vi "ImagerForFlowbit3.vi"() -> ()   [LabVIEW 2011]
uses:
  <vilib>/vision/Image Controls.llb/IMAQ Image.ctl
  <vilib>/Platform/TimedLoop/XDataNode/timing_clust.ctl
  <vilib>/Platform/TimedLoop/XDataNode/nitl_modes.ctl
  <vilib>/Platform/TimedLoop/XDataNode/wakeup.ctl
  <vilib>/Analysis/1siggen.llb/Riffle Array (I32).vi
  <vilib>/Platform/TimedLoop/XDataNode/XDataNode.xnode
  <vilib>/Analysis/NI_AALBase.lvlib
  <vilib>/vision/NI_Vision_Development_Module.lvlib
  <vilib>/Platform/TimedLoop/XDataNode/XDNodeRunTimeDep.lvlib
panel:
  out "数组 2":bool[](array[boolean])
  out "OnlineMap Array":T1[](array[typedef])
  out "DR/R array":T1[](array[typedef])
  out "停止循环":bool
  in  "Stimuli":i64=5
  in  "FrameHeight":i64=576
  in  "FrameWidth":i64=704
  in  "选项卡控件":enum32{"前面板", "参数设置", "OnLineMap"}(tab)
  out "log":string
  out "Stim_ID":i32(listbox)=1
  in  "开始/暂停":bool=TRUE
  in  "停止":bool
  out "重排的 Stim ID":i32[](array[numeric]) caption="重排的{X}"
  out "block":i32
  out "队列中元素数量":i32
  out "Image 2":T1(plugin-control)
  in  "热图":bool
  out "循环持续时间":i64
  out "Recording":bool
  in  "FramesPerStim(100Hz)":i64=16
  in  "Blk目录":path=path "D:/Expt/test"
  in  "文件名":string="G4_E01"
  in  "TimeForPrepare(ms)":u32=1000
  in  "stim ID":u8[](array[numeric])=[0, 2, 4, 6, 8]
  in  "blk总数":i32=500
  in  "stim protocol":T2(array[ring])=[enum."prep stim", enum."wait respirator", enum."show stim", enum."recording data", enum."Blank stim", enum."ISI"]
  in  "blank stim":u8
  in  "wait（ms）":u32=10
  in  "ISI（ms）":u32=8000
  in  "FrameBin":i32=25
  in  "datatype":u16(ring)=13 items=["U8"=11, "I16"=12, "U32"=13, "SGL"=14]
  in  "OnlineMap":cluster{"数组 1":i32[], "数组 2":i32[]}[](array[cluster])=[{"数组 1"=[2], "数组 2"=[6]}, {"数组 1"=[4], "数组 2"=[8]}, {"数组 1"=[2, 6], "数组 2"=[4, 8]}, {"数组 1"=[2, 4, 6, 8], "数组 2"=[0]}, {"数组 1"=[2, 4], "数组 2"=[6, 8]}]
  in  "DR/R parameter":T3={"frame_zero_0"=0, "frame_zero_1"=1, "frame_0"=3, "frame_1"=15}
  # "÷"
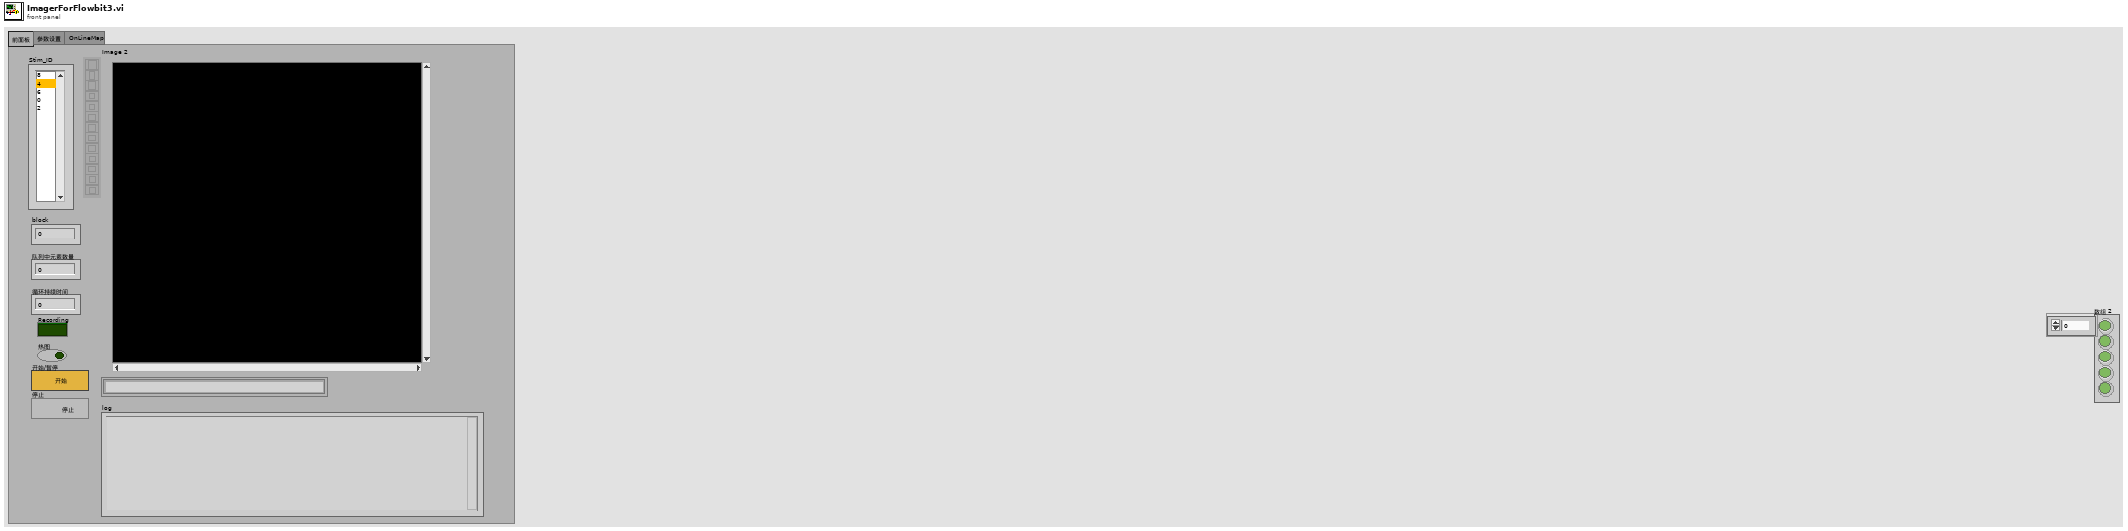
[diagram p1: front panel]
types:
  T1 = typedef "IMAQ Image.ctl" = refnum<image>
  T2 = enum16{"wait", "prep stim", "show stim", "wait respirator", "recording data", "Blank stim", "wait heart", "ISI", "DR/R", "wait calibrate"}[]
  T3 = cluster{"frame_zero_0":i32, "frame_zero_1":i32, "frame_0":i32, "frame_1":i32}
  T4 = typedef "Image Type" = u32
  T5 = enum16{"Disable External Trigger", "Enable External Trigger"}
  T6 = enum32{"Auto Detect", "RoadRunner", "Raven", "R64"}
  T7 = typedef "XDNodeRunTimeDep.lvlib/timing_clust.ctl" = cluster{"Expected End [f-1]":u64, "Actual End [f-1]":u64, "Finished Late? [f-1]":bool, "Expected End [i-1]":u64, "Actual End [i-1]":u64, "Finished Late? [i-1]":bool, "Expected Start [i]":u64, "Actual Start [i]":u64, "Expected Start [f]":u64, "Actual Start [f]":u64, "Source Name":string, "Structure Name":string, "Period":i64, "Deadline":i64, "Offset":i64, "Start":i64, "Priority":i32, "Timeout":i32, "Mode":T8, "Wakeup Reason":T9, "Error":errorcluster, "Source Type":string, "Secondary Source Type":string, "Global End Time":u64, "Global Start Time":u64, "Frame Duration":u64, "Iteration Duration":u64, "Assigned CPU":i32, "I/O Scan Engine Mode":u32}
  T8 = typedef "XDNodeRunTimeDep.lvlib/nitl_modes.ctl" = enum32{"No Change", "Process missed periods, maintain original phase", "Discard missed periods, maintain original phase", "Process missed periods, ignore original phase", "Discard missed periods, ignore original phase"}
  T9 = typedef "XDNodeRunTimeDep.lvlib/wakeup.ctl" = enum32{"Normal", "Aborted", "Asynchronous wakeup", "Timing source error", "Timed loop error", "Timeout"}
  T10 = enum16{"big-endian, network order", "native, host order", "little-endian"}
  T11 = enum16{"open", "replace", "create", "open or create", "replace or create", "replace or create with confirmation"}
  T12 = cluster{"Mean Value":sgl, "Standard Variation":sgl, "Minimal Value":sgl, "Maximal Value":sgl, "Area (calibrated)":sgl, "Area (pixels)":u32, "%":sgl, "Calibration Valid":bool}
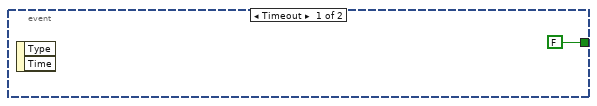
[diagram p2: hidden frame]
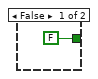
[diagram p3: hidden frame]
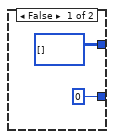
[diagram p5: hidden frame]
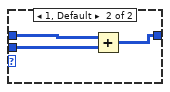
[diagram p7: hidden frame]
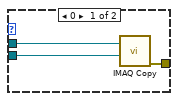
[diagram p8: hidden frame]
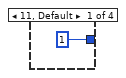
[diagram p9: hidden frame]
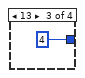
[diagram p10: hidden frame]
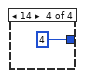
[diagram p11: hidden frame]
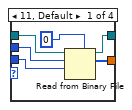
[diagram p12: hidden frame]
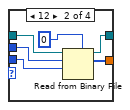
[diagram p13: hidden frame]
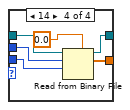
[diagram p14: hidden frame]
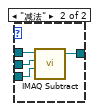
[diagram p18: hidden frame]
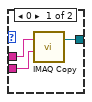
[diagram p19: hidden frame]
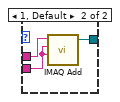
[diagram p20: hidden frame]
diagram:
  w1 = u32[][] []
  w14 = T4 4 items=["Grayscale (U8)", "Grayscale (I16)", "Grayscale (SGL)", "Complex (CSG)", "RGB (U32)", "HSL (U32)", "RGB (U64)", "Grayscale (U16)"] ("Image Type")
  w12 = u32[] [160, 240, 2105599, 873983, 50382, 65535, 65344, 8454016, 16776960, 16777088, 16744512, 16711680, 16711935, 8388863, 5111914, 16777222, 16448250] ("数组")
  w18 = T4 1 items=["Grayscale (U8)", "Grayscale (I16)", "Grayscale (SGL)", "Complex (CSG)", "RGB (U32)", "HSL (U32)", "RGB (U64)", "Grayscale (U16)"] ("Image Type")
  w20 = T4 1 items=["Grayscale (U8)", "Grayscale (I16)", "Grayscale (SGL)", "Complex (CSG)", "RGB (U32)", "HSL (U32)", "RGB (U64)", "Grayscale (U16)"] ("Image Type")
  n1 = flat-sequence {
    tunnel: [TRUE ("Zoom to Fit Mode")] -> w5
    frame #0 {
      w55 = T4 0 items=["Grayscale (U8)", "Grayscale (I16)", "Grayscale (SGL)", "Complex (CSG)", "RGB (U32)", "HSL (U32)", "RGB (U64)", "Grayscale (U16)"] ("Image Type")
      w58 = T4 2 items=["Grayscale (U8)", "Grayscale (I16)", "Grayscale (SGL)", "Complex (CSG)", "RGB (U32)", "HSL (U32)", "RGB (U64)", "Grayscale (U16)"] ("Image Type")
      # "DB25\tU32顺序\tport\tread/write\t反转逻辑\n1\t     16\t   p2.0    \tW\t        是\n2\t     0    \tp0.0\t   \tR&W\t      否\n3\t     1\t\t   p0.1\t   \tR&W      \t否\n4\t\t    2\t   \tp0.2   \t\tR&W      \t否\n5\t\t    3\t\t   p0.3   \t\tR&W\t      否\n6\t\t    4\t   \tp0.4   \t\tR&W      \t否\n7\t\t    5\t   \tp0.5   \t\tR&W      \t否\n8\t\t    6\t   \tp0.6\t   \tR&W      \t否\n9\t    \t7\t   \tp0.7\t   \tR&W\t      否\n10\t    14   \tp1.3   \t\tR        \t否\n11\t   \t15   \tp1.4   \t\tR        \t是\n12\t   \t13   \tp1.2\t   \tR        \t否\n13    \t12   \tp1.1\t   \tR        \t否\n14     17   \tp2.1\t   \tW        \t是\n15    \t11   \tp1.0   \t\tR\t        否\n16    \t18   \tp2.2   \t\tW        \t否\n17    \t19\t   p2.3   \t\tW\t        是\n18    \t20   \tN   \t  \tGND\t\n19    \t21   \tN   \t  \tGND\t\n20\t    22\t   N\t  \t  \tGND\t\n21\t    23\t   N  \t  \t\tGND\t\n22\t    24\t   N  \t  \t\tGND\t\n23    \t10   \tN  \t  \t\tGND\t\n24    \t9\t    N  \t  \t\tGND\t\n25\t    8    \tN  \t  \t\tGND"
      n2 = local write "停止循环"(FALSE ("开始/暂停")) -> ()
      n3 = local write "开始/暂停"(TRUE ("开始/暂停")) -> ()
      n4 = call "Set_para_port0.vi"("R or W"=enum16{"read", "write"}."write") -> ()  [unwired: 9 in, 2 out]
      n5 = call "IMAQ Create"("Image Name"="write file data", "Image Type"=w55) -> ()  [unwired: 3 in, 2 out]
      n6 = call "IMAQ Create"("Image Name"="OnlineMap temp2", "Image Type"=w58) -> ()  [unwired: 3 in, 2 out]
      n7 = call "IMAQ Create"("Image Name"="OnlineMap temp1", "Image Type"=w58) -> ()  [unwired: 3 in, 2 out]
    }
  }
  n8 = local write "Recording"(FALSE ("Recording")) -> ()
  n9 = call <vilib>:"open.vi"("Board Type"=T6."Auto Detect", "Board Number"=u32 0) -> ("error out"=w36:errorcluster, "RefBrdOut"=w31:u32)  [unwired: 2 in, 5 out]
  n10 = call <vilib>:"New Image.vi"("RefBrdIn"=w31, "error in"=w36) -> ("RefBrdOut"=w30:u32, "Image"=w45:T1, "error out"=w37:errorcluster)  [unwired: 6 in]
  n11 = call <vilib>:"Trigger Mode.vi"("RefBrdIn"=w30, "Trigger Mode"=T5."Disable External Trigger", "error in (no error)"=w37) -> ("RefBrdOut"=w29:u32, "error out"=w38:errorcluster)  [unwired: 6 in]
  n12 = call <vilib>:"Setup.vi"("error in"=w38, "Image In"=w45, "RefBrdIn"=w29) -> ("error out"=w33:errorcluster, "Image"=w34:T1, "RefBrdOut"=w28:u32)  [unwired: 6 in]
  n13 = Obtain Queue(name (unnamed)="FrameQueue" ("名称（未命名）"), element data type=w1) -> (queue out=w8:refnum<queue>)  [unwired: 3 in, 2 out]
  n14 = call "IMAQ Create"("Image Name"="recording", "Image Type"=w20) -> ("New Image"=w22:T1)  [unwired: 3 in, 1 out]
  n15 = call "IMAQ Create"("Image Name"="display", "Image Type"=w18) -> ("New Image"=w16:T1)  [unwired: 3 in, 1 out]
  n16 = call "IMAQ Create"("Image Name"="display2", "Image Type"=w14) -> ("New Image"=w13:T1)  [unwired: 3 in, 1 out]
  n17 = Type Cast(type=sgl[] [] ("单精度浮点"), x=w12) -> (*(type *) &x=w10:sgl[])
  n18 = call <vilib>:"Continuous Grab.vi"("error in (no error)"=w33, "Image In"=w34, "RefBrdIn"=w28) -> ("error out"=w32:errorcluster, "Image"=w19:T1, "RefBrdOut"=w27:u32)  [unwired: 6 in]
  n19 = Flush Queue(queue=w8) -> (queue out=w2:refnum<queue>)  [unwired: 1 in, 2 out]
  n20 = call "IMAQ GetImageInfo"("Image"=w19) -> ("Y Resolution"=w6:i32, "X Resolution"=w7:i32)  [unwired: 3 in, 6 out]
  n21 = node-c288() -> (w49:T7)
  n22 = local write "FrameWidth"(w7) -> ()
  n23 = local write "FrameHeight"(w6) -> ()
  n24 = while {
    tunnel: "stim ID" -> [w72]
    tunnel: "文件名" -> [w71]
    tunnel: "Blk目录" -> [w70]
    tunnel: w5 -> [_]
    tunnel: w2 -> [w63]
    stop <- w68 stop-if-true
    n25 = Wait (ms)(milliseconds to wait=u32 200 ("等待时间（毫秒）")) -> ()  [unwired: 1 out]
    n26 = local read "开始/暂停"() -> (w67:bool)
    n27 = Select(t=0, s=w67, f="blk总数") -> (s? t:f=w64:i32)
    n28 = for {
      N: w64 -> [_]
      tunnel: w72 -> [w79]
      tunnel: w71 -> [w87]
      tunnel: w70 -> [w86]
      tunnel: w63 -> [w73]
      i -> [w74]
      stop <- w80 stop-if-true
      # "block循环"
      n29 = flat-sequence {
        tunnel: [w333] -> w84
        tunnel: [w332] -> w78
        tunnel: w74 -> [w331]
        tunnel: w87 -> [w338]
        tunnel: w86 -> [w334]
        tunnel: w79 -> [w332]
        tunnel: w84 -> [w395]
        tunnel: [w395] -> w83
        tunnel: [w393] -> w82
        tunnel: w78 -> [w392]
        tunnel: [w391] -> w77
        tunnel: w83 -> [w406]
        tunnel: [w408] -> w85
        tunnel: w82 -> [w407]
        tunnel: [w407] -> w81
        tunnel: w77 -> [w396]
        tunnel: [w396] -> w76
        frame #0 {
          # "创建onlinemap所需要的空间"
          # "创建文件名"
          n30 = Number To Decimal String(number=w331, width (-)=i16 3 ("宽度(-)")) -> ()  [unwired: 1 out]
          n31 = Number To Decimal String(number=w331, width (-)=i16 3 ("宽度(-)")) -> (decimal integer string=w340:string)
          n32 = call <vilib>:"Space Constant.vi"() -> ("String"=w341:string)
          n33 = case shown="0" w331 {
            tunnel: w332 -> [_ w350]
            frame 1, Default {
            }
            frame 0 {
              n34 = for {
                tunnel: w350 -> [w387] mode=indexing
                tunnel: [w384] -> w349 mode=indexing
                w390 = T4 2 items=["Grayscale (U8)", "Grayscale (I16)", "Grayscale (SGL)", "Complex (CSG)", "RGB (U32)", "HSL (U32)", "RGB (U64)", "Grayscale (U16)"] ("Image Type")
                n35 = Number To Decimal String(number=w387) -> (decimal integer string=w388:string)  [unwired: 1 in]
                n36 = Concatenate Strings("Stim", w388, "_DR/R" ("字符串")) -> (w385:string)
                n37 = call "IMAQ Create"("Image Name"=w385, "Image Type"=w390) -> ("New Image"=w384:T1)  [unwired: 3 in, 1 out]
              }
              "DR/R array" <- w349
              n38 = for {
                tunnel: "OnlineMap" -> [w361] mode=indexing
                tunnel: [w351] -> w347 mode=indexing
                w359 = T4 2 items=["Grayscale (U8)", "Grayscale (I16)", "Grayscale (SGL)", "Complex (CSG)", "RGB (U32)", "HSL (U32)", "RGB (U64)", "Grayscale (U16)"] ("Image Type")
                n39 = Unbundle By Name(w361) -> ("数组 1"=w360:i32[], "数组 2"=w356:i32[])
                n40 = for {
                  tunnel: w360 -> [w376] mode=indexing
                  shift-right: [w374] -> w357
                  shift-left: "" -> [w373]
                  i -> [w378]
                  n41 = Number To Decimal String(number=w376) -> (decimal integer string=w375:string)  [unwired: 1 in]
                  n42 = Equal To 0?(x=w378) -> (x = 0?=w377:bool)
                  n43 = case shown="假" w377 {
                    tunnel: w375 -> [w379 w383]
                    tunnel: [w382 w383] -> w374
                    tunnel: w373 -> [w381 _]
                    frame False {
                      n44 = Concatenate Strings(w381, "+" ("字符串"), w379) -> (w382:string)
                    }
                    frame True {
                    }
                  }
                }
                n45 = for {
                  tunnel: w356 -> [w365] mode=indexing
                  shift-right: [w363] -> w354
                  shift-left: "" -> [w362]
                  i -> [w367]
                  n46 = Number To Decimal String(number=w365) -> (decimal integer string=w364:string)  [unwired: 1 in]
                  n47 = Equal To 0?(x=w367) -> (x = 0?=w366:bool)
                  n48 = case shown="假" w366 {
                    tunnel: w364 -> [w368 w372]
                    tunnel: [w371 w372] -> w363
                    tunnel: w362 -> [w370 _]
                    frame False {
                      n49 = Concatenate Strings(w370, "+" ("字符串"), w368) -> (w371:string)
                    }
                    frame True {
                    }
                  }
                }
                n50 = Concatenate Strings(w357, "/" ("字符串"), w354) -> (w352:string)
                n51 = call "IMAQ Create"("Image Name"=w352, "Image Type"=w359) -> ("New Image"=w351:T1)  [unwired: 3 in, 1 out]
              }
              "OnlineMap Array" <- w347
            }
          }
          n52 = Search and Replace String(replace all?=TRUE ("替换全部？(F)"), input string=w340, search string=w341, replace string="0" ("替换字符串(\"\")")) -> (result string=w337:string)  [unwired: 4 in, 3 out]
          n53 = for {
            tunnel: string[] ["Temp_DR/R", "frame_zero", "Mean_frame_zero", "frame", "Mean_frame", "Temp_DR", "Empty"] ("添加的数组") -> [w345] mode=indexing
            w346 = T4 2 items=["Grayscale (U8)", "Grayscale (I16)", "Grayscale (SGL)", "Complex (CSG)", "RGB (U32)", "HSL (U32)", "RGB (U64)", "Grayscale (U16)"] ("Image Type")
            n54 = call "IMAQ Create"("Image Name"=w345, "Image Type"=w346) -> ()  [unwired: 3 in, 2 out]
          }
          n55 = Concatenate Strings(w338, w337, ".blk" ("字符串")) -> (w335:string)
          n56 = Build Path(base path=w334, name or relative path=w335) -> (appended path=w333:path)
        }
        frame #1 {
          # "random ID"
          n57 = call-poly <vilib>:"Riffle.vi"("X"=w392) -> ("Riffled Index"=w391:i32[], "Riffled {X}"=w393:i32[])  [unwired: 8 in, 1 out]
          "重排的 Stim ID" <- w393
          n58 = Number To Decimal String(number=w393) -> (decimal integer string=w394:string[])  [unwired: 1 in]
          n59 = property on="Stim_ID" class="LstBox (严格)"("Item Names"=w394) -> ()  [unwired: 2 in, 2 out]
        }
        frame #2 {
          # "写头文件"
          n60 = local read "FrameHeight"() -> (w398:i64)
          n61 = local read "FrameWidth"() -> (w397:i64)
          n62 = Initialize Array(sgl 0.0 ("元素"), w398, w397) -> (w402:sgl[][])
          n63 = call "IMAQ ArrayToImage"("Image Pixels (Float)"=w402, "Image"="Mean_frame" ("Image Name")) -> ()  [unwired: 8 in, 2 out]
          n64 = call "IMAQ ArrayToImage"("Image Pixels (Float)"=w402, "Image"="Mean_frame_zero" ("Image Name")) -> ()  [unwired: 8 in, 2 out]
          n65 = Open/Create/Replace File(file path (use dialog)=w406, operation (0:open)=T11."open or create" ("操作(0:open)")) -> (refnum out=w404:refnum<file>)  [unwired: 4 in, 2 out]
          n66 = call "BlkHeadWrite.vi"("SequenceOfID"=w407, "Stimuli"="Stimuli", "FramesPerStim"="FramesPerStim(100Hz)", "datatype"="datatype", "FrameHeight"="FrameHeight", "FrameWidth"="FrameWidth", "BlkFile"=w404) -> ("引用句柄输出"=w408:refnum<file>)  [unwired: 4 in]
        }
      }
      n67 = for {
        tunnel: w85 -> [w421]
        tunnel: [w419] -> w75
        tunnel: w76 -> [w420] mode=indexing
        tunnel: w81 -> [w418] mode=indexing
        tunnel: [w417] -> w80
        tunnel: w74 -> [w414]
        tunnel: w73 -> [w413]
        i -> [w416]
        stop <- w417 stop-if-true
        # "stim循环"
        n68 = for {
          tunnel: w420 -> [w428]
          tunnel: w418 -> [w426]
          tunnel: [w424] -> w417
          tunnel: "stim protocol" -> [w425] mode=indexing
          tunnel: w421 -> [w429]
          tunnel: [w427] -> w419
          tunnel: w414 -> [w423]
          tunnel: w413 -> [w422]
          stop <- w424 stop-if-true
          n69 = case shown="\"recording data\"" w425 {
            tunnel: w429 -> [w432 w449 w463 w478 w554 w567 w581 w596 w618]
            tunnel: w428 -> [_ _ _ w477 _ _ _ w594 _]
            tunnel: [w432 w449 w463 w476 w554 w567 w581 w596 w618] -> w427
            tunnel: w426 -> [w430 _ _ _ _ _ _ _ _]
            tunnel: [w433 w450 w464 w479 w555 w568 w582 w595 w619] -> w424
            tunnel: w423 -> [_ _ _ _ _ _ _ w593 _]
            tunnel: w422 -> [_ _ _ w474 _ _ _ _ _]
            frame "prep stim" {
              n70 = Number To Boolean Array(number=w430) -> (Boolean array=w434:bool[])
              n71 = flat-sequence {
                tunnel: w434 -> [w445]
                tunnel: [w445] -> w431
                tunnel: w430 -> [w444]
                tunnel: w431 -> [w447]
                frame #0 {
                  n72 = Number To Decimal String(number=w444) -> (decimal integer string=w441:string)  [unwired: 1 in]
                  n73 = Format Date/Time String() -> (date/time string=w443:string)  [unwired: 3 in]
                  n74 = local read "log"() -> (w437:string)
                  n75 = Concatenate Strings(w443, "\t", "prep stim ID=" ("字符串"), w441, "\r", w437) -> (w439:string)
                  n76 = String Subset(string=w439, length (rest)=1000 ("y")) -> (substring=w438:string)  [unwired: 1 in]
                  n77 = local write "log"(w438) -> ()
                }
                frame #1 {
                  n78 = call "Write_para_port0.vi"("port0（8元素）"=w447) -> ()  [unwired: 10 in, 1 out]
                  n79 = call "Write_para_port2.vi"("port2（4元素）"=bool[] [TRUE, FALSE, FALSE, FALSE] ("port2")) -> ()  [unwired: 10 in, 1 out]
                }
                frame #2 {
                  n80 = Wait (ms)(milliseconds to wait="TimeForPrepare(ms)") -> ()  [unwired: 1 out]
                }
              }
              n81 = local read "开始/暂停"() -> (w433:bool)
            }
            frame "wait respirator" {
              n82 = while {
                stop <- w460 stop-if-true
                n83 = call "read_para_port1.vi"() -> ("port1（5元素）"=w462:bool[])  [unwired: 10 in, 1 out]
                n84 = Index Array(array=w462, index=3 ("索引")) -> (element=w460:bool)
                n85 = Wait (ms)(milliseconds to wait=u32 5 ("等待时间（毫秒）")) -> ()  [unwired: 1 out]
              }
              n86 = flat-sequence {
                frame #0 {
                  n87 = Format Date/Time String() -> (date/time string=w458:string)  [unwired: 3 in]
                  n88 = local read "log"() -> (w453:string)
                  n89 = Concatenate Strings(w458, "\t", "wait respiratory" ("字符串"), "\r", w453) -> (w455:string)
                  n90 = String Subset(string=w455, length (rest)=1000 ("y")) -> (substring=w454:string)  [unwired: 1 in]
                  n91 = local write "log"(w454) -> ()
                }
              }
              n92 = local read "开始/暂停"() -> (w450:bool)
            }
            frame "show stim" {
              n93 = flat-sequence {
                frame #0 {
                  n94 = call "Write_para_port2.vi"("port2（4元素）"=bool[] [FALSE, FALSE, FALSE, FALSE] ("port2")) -> ()  [unwired: 10 in, 1 out]
                }
              }
              n95 = flat-sequence {
                frame #0 {
                  n96 = Format Date/Time String() -> (date/time string=w472:string)  [unwired: 3 in]
                  n97 = local read "log"() -> (w467:string)
                  n98 = Concatenate Strings(w472, "\t", "show stim" ("字符串"), "\r", w467) -> (w469:string)
                  n99 = String Subset(string=w469, length (rest)=1000 ("y")) -> (substring=w468:string)  [unwired: 1 in]
                  n100 = local write "log"(w468) -> ()
                }
              }
              n101 = local read "开始/暂停"() -> (w464:bool)
            }
            frame "recording data" {
              n102 = flat-sequence {
                frame #0 {
                  n103 = Format Date/Time String() -> (date/time string=w491:string)  [unwired: 3 in]
                  n104 = local read "log"() -> (w486:string)
                  n105 = Concatenate Strings(w491, "\t", "recording data" ("字符串"), "\r", w486) -> (w488:string)
                  n106 = String Subset(string=w488, length (rest)=1000 ("y")) -> (substring=w487:string)  [unwired: 1 in]
                  n107 = local write "log"(w487) -> ()
                }
              }
              n108 = local read "FramesPerStim(100Hz)"() -> (w480:i64)
              n109 = for {
                N: w480 -> [_]
                tunnel: ["开始/暂停"] -> w479
                tunnel: w478 -> [w518]
                tunnel: w477 -> [w500]
                tunnel: [w509] -> w476
                tunnel: [w508] -> w475
                tunnel: w474 -> [w492]
                i -> [w498]
                stop <- "开始/暂停" stop-if-true
                n110 = Get File Size(file=w518) -> (refnum out=w510:refnum<file>, size (in bytes)=w505:i64)  [unwired: 1 in, 1 out]
                n111 = local read "datatype"() -> (w513:u16)
                n112 = case shown="13" w513 {
                  tunnel: [i64 1 i64 2 i64 4 i64 4] -> w504
                  frame 11, Default {
                  }
                  frame 12 {
                  }
                  frame 13 {
                  }
                  frame 14 {
                  }
                }
                n113 = local read "FramesPerStim(100Hz)"() -> (w501:i64)
                n114 = local read "FrameHeight"() -> (w502:i64)
                n115 = local read "FrameWidth"() -> (w503:i64)
                n116 = Multiply(x=w501, y=w500) -> (x*y=w499:i64)
                n117 = Add(x=w499, y=w498) -> (x+y=w497:i64)
                n118 = Compound Arithmetic op=MULTIPLY(w504, w503, w502) -> (w496:i64)
                n119 = Multiply(x=w496, y=w497) -> (x*y=w495:i64)
                n120 = Add(x=w495, y=i64 1716 ("x")) -> (x+y=w493:i64)
                n121 = Greater?(x=w493, y=w505) -> (0:w511:bool)
                n122 = case shown="真" w511 {
                  tunnel: w493 -> [_ w549]
                  tunnel: w510 -> [w546 w548]
                  tunnel: [w546 w547] -> w512
                  frame False {
                  }
                  frame True {
                    n123 = Set File Size(6:w549, 7:w548) -> (3:w547:refnum<file>)  [unwired: 1 in, 1 out]
                  }
                }
                n124 = Dequeue Element(queue=w492, timeout in ms (-1)=4000 ("超时毫秒(-1)")) -> (queue out=w508:refnum<queue>, element=w507:u32[][])  [unwired: 1 in, 2 out]
                n125 = Set File Position(offset (in bytes) (0)=w493, refnum=w512) -> (refnum out=w516:refnum<file>, error out=w514:errorcluster)  [unwired: 2 in]
                n126 = case shown="14" w513 {
                  tunnel: w507 -> [w521 w528 w533 w539]
                  tunnel: w516 -> [w525 w529 w536 w541]
                  tunnel: T10."native, host order" ("字节顺序(0:big-endian, network order)") -> [w524 w530 w534 w542]
                  tunnel: w514 -> [w523 _ w535 w543]
                  tunnel: [w522 w531 w537 w544] -> w509
                  frame 11, Default {
                    n127 = To Unsigned Byte Integer(number=w521) -> (unsigned 8bit integer=w520:u8[][])
                    n128 = Write to Binary File(file (use dialog)=w525, data=w520, error in=w523, 5:FALSE ("预置数组或字符串大小？(T)"), 9:w524) -> (refnum out=w522:refnum<file>)  [unwired: 1 in, 2 out]
                  }
                  frame 12 {
                    n129 = To Unsigned Word Integer(number=w528) -> (unsigned 16bit integer=w527:u16[][])
                    n130 = Write to Binary File(file (use dialog)=w529, data=w527, 5:FALSE ("预置数组或字符串大小？(T)"), 9:w530) -> (refnum out=w531:refnum<file>)  [unwired: 2 in, 2 out]
                  }
                  frame 13 {
                    n131 = Write to Binary File(file (use dialog)=w536, data=w533, error in=w535, 5:FALSE ("预置数组或字符串大小？(T)"), 9:w534) -> (refnum out=w537:refnum<file>)  [unwired: 1 in, 2 out]
                  }
                  frame 14 {
                    n132 = To Single Precision Float(number=w539) -> (single precision float=w540:sgl[][])
                    n133 = Write to Binary File(file (use dialog)=w541, data=w540, error in=w543, 5:FALSE ("预置数组或字符串大小？(T)"), 9:w542) -> (refnum out=w544:refnum<file>)  [unwired: 1 in, 2 out]
                  }
                }
                "Recording" <- TRUE ("Recording")
              }
              n134 = flat-sequence {
                tunnel: w475 -> [w482]
                frame #0 {
                  n135 = Flush Queue(queue=w482) -> ()  [unwired: 1 in, 3 out]
                  n136 = local write "Recording"(FALSE ("Recording")) -> ()
                  n137 = Request Deallocation(TRUE ("标志")) -> ()
                }
              }
            }
            frame "Blank stim" {
              n138 = flat-sequence {
                frame #0 {
                  n139 = Format Date/Time String() -> (date/time string=w565:string)  [unwired: 3 in]
                  n140 = local read "log"() -> (w560:string)
                  n141 = Concatenate Strings(w565, "\t", "show blank stim" ("字符串"), "\r", w560) -> (w562:string)
                  n142 = String Subset(string=w562, length (rest)=1000 ("y")) -> (substring=w561:string)  [unwired: 1 in]
                  n143 = local write "log"(w561) -> ()
                }
              }
              n144 = Number To Boolean Array(number="blank stim") -> (Boolean array=w556:bool[])
              n145 = call "Write_para_port0.vi"("port0（8元素）"=w556) -> ()  [unwired: 10 in, 1 out]
              n146 = local read "开始/暂停"() -> (w555:bool)
            }
            frame "ISI" {
              n147 = flat-sequence {
                tunnel: "ISI（ms）" -> [w572]
                tunnel: "ISI（ms）" -> [w579]
                frame #0 {
                  n148 = Number To Decimal String(number=w572) -> (decimal integer string=w576:string)  [unwired: 1 in]
                  n149 = Format Date/Time String() -> (date/time string=w578:string)  [unwired: 3 in]
                  n150 = local read "log"() -> (w571:string)
                  n151 = Concatenate Strings(w578, "\t", "ISI(ms)=" ("字符串"), w576, "\r", w571) -> (w574:string)
                  n152 = String Subset(string=w574, length (rest)=1000 ("y")) -> (substring=w573:string)  [unwired: 1 in]
                  n153 = local write "log"(w573) -> ()
                }
                frame #1 {
                  n154 = Wait (ms)(milliseconds to wait=w579) -> ()  [unwired: 1 out]
                }
              }
              n155 = local read "开始/暂停"() -> (w568:bool)
            }
            frame "wait", Default {
              n156 = Wait (ms)(milliseconds to wait="wait（ms）") -> ()  [unwired: 1 out]
              n157 = flat-sequence {
                tunnel: "wait（ms）" -> [w586]
                frame #0 {
                  n158 = Number To Decimal String(number=w586) -> (decimal integer string=w590:string)  [unwired: 1 in]
                  n159 = Format Date/Time String() -> (date/time string=w592:string)  [unwired: 3 in]
                  n160 = local read "log"() -> (w585:string)
                  n161 = Concatenate Strings(w592, "\t", "wait(ms)=" ("字符串"), w590, "\r", w585) -> (w588:string)
                  n162 = String Subset(string=w588, length (rest)=1000 ("y")) -> (substring=w587:string)  [unwired: 1 in]
                  n163 = local write "log"(w587) -> ()
                }
              }
              n164 = local read "开始/暂停"() -> (w582:bool)
            }
            frame "DR/R" {
              n165 = disable-structure shown="禁用" {
                frame Disabled {
                  n166 = flat-sequence {
                    frame #0 {
                      n167 = Format Date/Time String() -> (date/time string=w604:string)  [unwired: 3 in]
                      n168 = local read "log"() -> (w599:string)
                      n169 = Concatenate Strings(w604, "\t", "DR/R" ("字符串"), "\r", w599) -> (w601:string)
                      n170 = String Subset(string=w601, length (rest)=1000 ("y")) -> (substring=w600:string)  [unwired: 1 in]
                      n171 = local write "log"(w600) -> ()
                    }
                  }
                }
                frame Enabled {
                }
              }
              n172 = disable-structure shown="禁用" {
                disable-tunnel: w594 -> [w609 _]
                disable-tunnel: w593 -> [w608 _]
                frame Disabled {
                  n173 = local read "DR/R array"() -> (w605:T1[])
                  n174 = Index Array(array=w605, index=w609) -> (element=w606:T1)
                  n175 = call "dR.vi"() -> ("Image Dst Out"=w607:T1)  [unwired: 11 in]
                  n176 = case shown="0" w608 {
                    selector: w608 -> [_ w614]
                    tunnel: w607 -> [w611 w615]
                    tunnel: w606 -> [w610 w617]
                    frame 0 {
                      n177 = call "IMAQ Copy"("Image Dst"=w610, "Image Src"=w611) -> ()  [unwired: 4 in, 2 out]
                    }
                    frame 1, Default {
                      n178 = Increment(x=w614) -> (x+1=w613:i32)
                      n179 = call "IMAQ Multiply"("Image Src A"=w617, "Constant"=w614, "Image Dst"=w617) -> ("Image Dst Out"=w616:T1)  [unwired: 4 in, 1 out]
                      n180 = call "IMAQ Add"("Image Src A"=w616, "Image Dst"=w616, "Image Src B"=w615) -> ("Image Dst Out"=w612:T1)  [unwired: 4 in, 1 out]
                      n181 = call "IMAQ Divide"("Image Src A"=w612, "Constant"=w613, "Image Dst"=w612) -> ()  [unwired: 4 in, 2 out]
                    }
                  }
                }
                frame Enabled {
                }
              }
              n182 = local read "开始/暂停"() -> (w595:bool)
            }
            frame "wait heart" {
              n183 = flat-sequence {
                frame #0 {
                  n184 = Format Date/Time String() -> (date/time string=w627:string)  [unwired: 3 in]
                  n185 = local read "log"() -> (w622:string)
                  n186 = Concatenate Strings(w627, "\t", "wait heart" ("字符串"), "\r", w622) -> (w624:string)
                  n187 = String Subset(string=w624, length (rest)=1000 ("y")) -> (substring=w623:string)  [unwired: 1 in]
                  n188 = local write "log"(w623) -> ()
                }
              }
              n189 = local read "开始/暂停"() -> (w619:bool)
            }
          }
        }
        "Stim_ID" <- w416
      }
      n190 = case shown="假" w80 {
        tunnel: w75 -> [w89 _]
        tunnel: w74 -> [w92 _]
        frame False {
          # "根据DR/R图计算onlinemap"
          n191 = local read "stim ID"() -> (w91:u8[])
          n192 = for {
            tunnel: w92 -> [w118]
            tunnel: w91 -> [_] mode=indexing
            tunnel: [w117] -> w90
            tunnel: w89 -> [w104]
            tunnel: [w99] -> w88
            i -> [w97]
            n193 = local read "FramesPerStim(100Hz)"() -> (w98:i64)
            n194 = Unbundle By Name("DR/R parameter") -> ("frame_zero_0"=w116:i32, "frame_zero_1"=w115:i32, "frame_0"=w113:i32, "frame_1"=w112:i32)
            n195 = local read "datatype"() -> (w100:u16)
            n196 = for {
              N: w98 -> [_]
              tunnel: w116 -> [w158]
              tunnel: w115 -> [w157]
              shift-right: [w163] -> _
              shift-left: 0 -> [w164]
              tunnel: w113 -> [w156]
              tunnel: w112 -> [w155]
              shift-right: [w161] -> _
              shift-left: 0 -> [w162]
              tunnel: [w159] -> w110 mode=indexing
              tunnel: w104 -> [w150]
              tunnel: "Mean_frame_zero" ("Image Name") -> [w153]
              tunnel: [w154] -> w120
              tunnel: "Mean_frame" ("Image Name") -> [w151]
              tunnel: [w152] -> w119
              tunnel: T10."native, host order" ("字节顺序(0:big-endian, network order)") -> [w148]
              tunnel: w100 -> [w144]
              tunnel: [w145] -> w99
              tunnel: w97 -> [w139]
              tunnel: w98 -> [w138]
              i -> [w136]
              n197 = case shown="12" w144 {
                tunnel: [i64 1 i64 2 i64 4 i64 4] -> w141
                frame 11, Default {
                }
                frame 12 {
                }
                frame 13 {
                }
                frame 14 {
                }
              }
              n198 = In Range and Coerce(upper limit=w157, x=w136, lower limit=w158) -> (In Range?=w159:bool)  [unwired: 1 out]
              n199 = In Range and Coerce(upper limit=w155, x=w136, lower limit=w156) -> (In Range?=w160:bool)  [unwired: 1 out]
              n200 = local read "FrameHeight"() -> (w142:i64)
              n201 = local read "FrameWidth"() -> (w140:i64)
              n202 = Compound Arithmetic op=ADD(w142, w141, w140) -> (w134:i64)
              n203 = Multiply(x=w138, y=w139) -> (x*y=w137:i64)
              n204 = Add(x=w136, y=w137) -> (x+y=w135:i64)
              n205 = Multiply(x=w135, y=w134) -> (x*y=w133:i64)
              n206 = Add(x=i64 1716, y=w133) -> (x+y=w131:i64)
              n207 = Multiply(x=w140, y=w142) -> (x*y=w143:i64)
              n208 = Set File Position(offset (in bytes) (0)=w131, refnum=w150) -> (refnum out=w149:refnum<file>)  [unwired: 2 in, 1 out]
              n209 = case shown="13" w144 {
                tunnel: w149 -> [w174 w179 w183 w191]
                tunnel: w143 -> [w173 w178 w185 w190]
                tunnel: w148 -> [w172 w177 w184 w189]
                tunnel: [w170 w176 w182 w188] -> w147
                tunnel: [w169 w175 w181 w187] -> w145
                frame 11, Default {
                  n210 = Read from Binary File(5:u8 0, 9:w172, 10:w173, 11:w174) -> (2:w170:u8[], 3:w169:refnum<file>)  [unwired: 2 in, 2 out]
                }
                frame 12 {
                  n211 = Read from Binary File(5:u16 0, 9:w177, 10:w178, 11:w179) -> (2:w176:u16[], 3:w175:refnum<file>)  [unwired: 2 in, 2 out]
                }
                frame 13 {
                  n212 = Read from Binary File(5:u32 0, 9:w184, 10:w185, 11:w183) -> (2:w182:u32[], 3:w181:refnum<file>)  [unwired: 2 in, 2 out]
                }
                frame 14 {
                  n213 = Read from Binary File(5:sgl 0.0, 9:w189, 10:w190, 11:w191) -> (2:w188:sgl[], 3:w187:refnum<file>)  [unwired: 2 in, 2 out]
                }
              }
              n214 = Reshape Array(w147, w142, w140) -> (w146:sgl[][])
              n215 = case shown="真" w159 {
                tunnel: w146 -> [_ w220]
                tunnel: w164 -> [w208 w219]
                tunnel: [w208 w215] -> w163
                tunnel: [w207 w210] -> w154
                tunnel: w153 -> [w207 w209]
                frame False {
                }
                frame True {
                  n216 = call "IMAQ ArrayToImage"("Image Pixels (Float)"=w220, "Image"="frame_zero" ("Image Name")) -> ("error out"=w216:errorcluster, "Image Out"=w211:T1)  [unwired: 8 in]
                  n217 = call "IMAQ Multiply"("Image Src A"=w209, "Constant"=w219, "Image Dst"=w209, "error in (no error)"=w216) -> ("Image Dst Out"=w212:T1, "error out"=w217:errorcluster)  [unwired: 3 in]
                  n218 = Increment(x=w219) -> (x+1=w215:i32)
                  n219 = call "IMAQ Add"("Image Src A"=w211, "Image Dst"=w212, "Image Src B"=w212, "error in (no error)"=w217) -> ("Image Dst Out"=w213:T1, "error out"=w218:errorcluster)  [unwired: 3 in]
                  n220 = call "IMAQ Divide"("Image Src A"=w213, "Constant"=w215, "Image Dst"=w213, "error in (no error)"=w218) -> ("Image Dst Out"=w210:T1)  [unwired: 3 in, 1 out]
                }
              }
              n221 = case shown="真" w160 {
                tunnel: w146 -> [_ w206]
                tunnel: w162 -> [w194 w204]
                tunnel: [w194 w198] -> w161
                tunnel: [w193 w196] -> w152
                tunnel: w151 -> [w193 w195]
                frame False {
                }
                frame True {
                  n222 = call "IMAQ ArrayToImage"("Image Pixels (Float)"=w206, "Image"="frame" ("Image Name")) -> ("error out"=w199:errorcluster, "Image Out"=w203:T1)  [unwired: 8 in]
                  n223 = call "IMAQ Multiply"("Image Src A"=w195, "Constant"=w204, "Image Dst"=w195, "error in (no error)"=w199) -> ("Image Dst Out"=w202:T1, "error out"=w200:errorcluster)  [unwired: 3 in]
                  n224 = Increment(x=w204) -> (x+1=w198:i32)
                  n225 = call "IMAQ Add"("Image Src A"=w203, "Image Dst"=w202, "Image Src B"=w202, "error in (no error)"=w200) -> ("Image Dst Out"=w197:T1, "error out"=w201:errorcluster)  [unwired: 3 in]
                  n226 = call "IMAQ Divide"("Image Src A"=w197, "Constant"=w198, "Image Dst"=w197, "error in (no error)"=w201) -> ("Image Dst Out"=w196:T1)  [unwired: 3 in, 1 out]
                }
              }
            }
            "数组 2" <- w110
            n227 = local read "DR/R array"() -> (w107:T1[])
            n228 = call "IMAQ Subtract"("Image Src A"=w120, "Image Dst"="Temp_DR" ("Image Name"), "Image Src B"=w119) -> ("Image Dst Out"=w105:T1)  [unwired: 4 in, 1 out]
            n229 = Index Array(array=w107, index=w97) -> (element=w106:T1)
            n230 = case shown="1, 默认" w118 {
              selector: w118 -> [_ w127]
              tunnel: w105 -> [w123 w128]
              tunnel: w106 -> [w122 w130]
              tunnel: [w121 w124] -> w117
              frame 0 {
                n231 = call "IMAQ Copy"("Image Dst"=w122, "Image Src"=w123) -> ("error out"=w121:errorcluster)  [unwired: 4 in, 1 out]
              }
              frame 1, Default {
                n232 = call "IMAQ Multiply"("Image Src A"=w130, "Constant"=w127, "Image Dst"=w130) -> ("Image Dst Out"=w129:T1)  [unwired: 4 in, 1 out]
                n233 = Increment(x=w127) -> (x+1=w126:i32)
                n234 = call "IMAQ Add"("Image Src A"=w129, "Image Dst"=w129, "Image Src B"=w128) -> ("Image Dst Out"=w125:T1)  [unwired: 4 in, 1 out]
                n235 = call "IMAQ Divide"("Image Src A"=w125, "Constant"=w126, "Image Dst"=w125) -> ("error out"=w124:errorcluster)  [unwired: 4 in, 1 out]
              }
            }
          }
          n236 = local read "OnlineMap Array"() -> (w95:T1[])
          n237 = local read "OnlineMap"() -> (w96:cluster{"数组 1":i32[], "数组 2":i32[]}[])
          n238 = Close File(refnum=w88) -> (error out=w93:errorcluster)  [unwired: 1 in, 1 out]
          n239 = for {
            tunnel: w96 -> [w275] mode=indexing
            tunnel: w95 -> [w266] mode=indexing
            tunnel: [w264] -> w94 mode=indexing
            tunnel: w90 -> [_]
            n240 = Unbundle By Name(w275) -> ("数组 1"=w274:i32[], "数组 2"=w269:i32[])
            n241 = flat-sequence {
              tunnel: w274 -> [w309]
              tunnel: [w308] -> w273
              tunnel: [w307] -> w272
              tunnel: w273 -> [w328]
              tunnel: w272 -> [w329]
              tunnel: [w327] -> w268
              frame #0 {
                n242 = Array Size(array=w309) -> (size(s)=w307:i32)
                n243 = for {
                  tunnel: w309 -> [w315] mode=indexing
                  tunnel: "OnlineMap temp1" ("Image Name") -> [w313]
                  tunnel: [w311] -> w308
                  i -> [w312]
                  n244 = flat-sequence {
                    tunnel: w315 -> [w324]
                    tunnel: [w322] -> w314
                    frame #0 {
                      n245 = Number To Decimal String(number=w324) -> (decimal integer string=w325:string)  [unwired: 1 in]
                      n246 = Concatenate Strings("Stim", w325, "_DR/R" ("字符串")) -> (w322:string)
                    }
                  }
                  n247 = case shown="0" w312 {
                    tunnel: w314 -> [w318 w321]
                    tunnel: w313 -> [w317 w320]
                    tunnel: [w316 w319] -> w311
                    frame 0 {
                      n248 = call "IMAQ Copy"("Image Dst"=w317, "Image Src"=w318) -> ("Image Dst Out"=w316:T1)  [unwired: 4 in, 1 out]
                    }
                    frame 1, Default {
                      n249 = call "IMAQ Add"("Image Src A"=w321, "Image Dst"=w320, "Image Src B"=w320) -> ("Image Dst Out"=w319:T1)  [unwired: 4 in, 1 out]
                    }
                  }
                }
              }
              frame #1 {
                n250 = call "IMAQ Divide"("Image Src A"=w328, "Constant"=w329, "Image Dst"=w328) -> ("Image Dst Out"=w327:T1)  [unwired: 4 in, 1 out]
              }
            }
            n251 = flat-sequence {
              tunnel: w269 -> [w286]
              tunnel: [w285] -> w271
              tunnel: [w284] -> w270
              tunnel: w271 -> [w305]
              tunnel: w270 -> [w306]
              tunnel: [w304] -> w267
              frame #0 {
                n252 = Array Size(array=w286) -> (size(s)=w284:i32)
                n253 = for {
                  tunnel: w286 -> [w292] mode=indexing
                  tunnel: "OnlineMap temp2" ("Image Name") -> [w290]
                  tunnel: [w288] -> w285
                  i -> [w289]
                  n254 = flat-sequence {
                    tunnel: w292 -> [w301]
                    tunnel: [w299] -> w291
                    frame #0 {
                      n255 = Number To Decimal String(number=w301) -> (decimal integer string=w302:string)  [unwired: 1 in]
                      n256 = Concatenate Strings("Stim", w302, "_DR/R" ("字符串")) -> (w299:string)
                    }
                  }
                  n257 = case shown="1, 默认" w289 {
                    tunnel: w291 -> [w295 w298]
                    tunnel: w290 -> [w294 w297]
                    tunnel: [w293 w296] -> w288
                    frame 0 {
                      n258 = call "IMAQ Copy"("Image Dst"=w294, "Image Src"=w295) -> ("Image Dst Out"=w293:T1)  [unwired: 4 in, 1 out]
                    }
                    frame 1, Default {
                      n259 = call "IMAQ Add"("Image Src A"=w298, "Image Dst"=w297, "Image Src B"=w297) -> ("Image Dst Out"=w296:T1)  [unwired: 4 in, 1 out]
                    }
                  }
                }
              }
              frame #1 {
                n260 = call "IMAQ Divide"("Image Src A"=w305, "Constant"=w306, "Image Dst"=w305) -> ("Image Dst Out"=w304:T1)  [unwired: 4 in, 1 out]
              }
            }
            n261 = case shown="\"除法\", 默认" enum16{"除法", "减法"}."除法" {
              tunnel: w268 -> [w277 w283]
              tunnel: w267 -> [w279 w282]
              tunnel: w266 -> [w276 w281]
              tunnel: [w278 w280] -> w264
              frame "除法", Default {
                n262 = call "IMAQ Divide"("Image Src A"=w277, "Image Dst"=w276, "Image Src B"=w279) -> ("Image Dst Out"=w278:T1)  [unwired: 4 in, 1 out]
              }
              frame "减法" {
                n263 = call "IMAQ Subtract"("Image Src A"=w283, "Image Dst"=w281, "Image Src B"=w282) -> ("Image Dst Out"=w280:T1)  [unwired: 4 in, 1 out]
              }
            }
          }
          n264 = call <vilib>:"Clear Errors.vi"("error in (no error)"=w93) -> ()  [unwired: 6 in, 1 out]
          n265 = for {
            tunnel: w94 -> [w251] mode=indexing
            i -> [w249]
            w235 = T4 0 items=["Grayscale (U8)", "Grayscale (I16)", "Grayscale (SGL)", "Complex (CSG)", "RGB (U32)", "HSL (U32)", "RGB (U64)", "Grayscale (U16)"] ("Image Type")
            n266 = case shown="真" TRUE {
              tunnel: [w252 w257] -> w230
              tunnel: w251 -> [w252 w256]
              frame False {
              }
              frame True {
                n267 = call "IMAQ Quantify 2"("Image"=w256) -> ("Global Report"=w263:T12)  [unwired: 8 in, 2 out]
                n268 = Unbundle By Name(w263) -> ("Mean Value"=w255:sgl, "Standard Variation"=w254:sgl)
                n269 = Multiply(x=w254, y=sgl 10.0) -> (x*y=w261:sgl)
                n270 = Subtract(x=w255, y=w261) -> (x-y=w260:sgl)
                n271 = Add(x=w255, y=w261) -> (x+y=w259:sgl)
                n272 = Bundle(w260, w259) -> (w258:cluster{sgl, sgl})  [unwired: 1 in]
                n273 = call "IMAQ Threshold"("Keep/Replace Value (Replace)"=TRUE, "Range"=w258, "Image Dst"=w256, "Image Src"=w256) -> ("Image Dst Out"=w257:T1)  [unwired: 6 in, 1 out]
              }
            }
            n274 = call "IMAQ WindZoom 2"("Window Number (0...15)"=w249, "Zoom Factor"=sgl 0.5) -> ("error out"=w231:errorcluster)  [unwired: 6 in, 3 out]
            n275 = call "IMAQ WindDraw"("Window Number (0...15)"=w249, "error in (no error)"=w231, "Title"=w230, "Image"=w230) -> ()  [unwired: 6 in, 2 out]
            n276 = call "IMAQ Quantify 2"("Image"=w230) -> ("Global Report"=w233:T12)  [unwired: 8 in, 2 out]
            n277 = Number To Decimal String(number=w249, width (-)=i16 2 ("宽度(-)")) -> (decimal integer string=w245:string)
            n278 = Unbundle By Name(w233) -> ("Maximal Value"=w232:sgl, "Minimal Value"=w229:sgl)
            n279 = call <vilib>:"Space Constant.vi"() -> ("String"=w244:string)
            n280 = local read "文件名"() -> (w247:string)
            n281 = Subtract(x=w232, y=w229) -> (x-y=w226:sgl)
            n282 = call "IMAQ Subtract"("Image Src A"=w230, "Constant"=w229) -> ("Image Dst Out"=w227:T1, "error out"=w228:errorcluster)  [unwired: 5 in]
            n283 = Search and Replace String(replace all?=TRUE ("替换全部？(F)"), input string=w245, search string=w244, replace string="0" ("替换字符串(\"\")")) -> (result string=w240:string)  [unwired: 4 in, 3 out]
            n284 = call "IMAQ Divide"("Image Src A"=w227, "Constant"=w226, "error in (no error)"=w228) -> ("Image Dst Out"=w224:T1, "error out"=w225:errorcluster)  [unwired: 4 in]
            n285 = local read "Blk目录"() -> (w238:path)
            n286 = Concatenate Strings(w247, "_" ("字符串"), w240, ".bmp" ("字符串")) -> (w237:string)
            n287 = call "IMAQ Multiply"("Image Src A"=w224, "Constant"=255, "error in (no error)"=w225) -> ("Image Dst Out"=w222:T1)  [unwired: 4 in, 1 out]
            n288 = call "IMAQ Cast Image"("Image Type"=w235, "Image Dst"="write file data" ("替换字符串(\"\")"), "Image Src"=w222) -> ("Image Dst Out"=w234:T1)  [unwired: 7 in, 1 out]
            n289 = Build Path(base path=w238, name or relative path=w237) -> (appended path=w236:path)
            n290 = call-poly "IMAQ Write File 2"("File Path"=w236, "Image"=w234) -> ()  [unwired: 8 in, 2 out]
          }
        }
        frame True {
        }
      }
      "block" <- w74
    }
    n291 = local read "停止循环"() -> (w68:bool)
  }
  n292 = Array Size(array="stim ID") -> (size(s)=w51:i32)
  n293 = timed-loop {
    tunnel: [w635] -> w44
    tunnel: [w649] -> w39
    tunnel: w19 -> [w635]
    tunnel: w32 -> [w648]
    tunnel: w27 -> [w647]
    tunnel: [w646] -> w26
    timing: w49 -> [_]
    timing-out: [_] -> w48
    tunnel: w22 -> [w636]
    tunnel: w2 -> [w630]
    tunnel: w16 -> [w641]
    tunnel: w12 -> [_]
    tunnel: w13 -> [w640]
    tunnel: w10 -> [w639]
    shift-right: [w633] -> _
    shift-left: 0 -> [w634]
    shift-right: [w632] -> _
    shift-left: w1 -> [w631]
    stop <- w642 stop-if-true
    n294 = node-c288() -> (→"循环持续时间":i64)  [unwired: 1 in]
    n295 = flat-sequence {
      tunnel: [w650] -> _
      frame #0 {
      }
      frame #1 {
        n296 = event shown="[1] \"停止\": 值改变" {
          selector: _ -> [_ _]
          dyn-events: _ -> [_ _]
          timeout: 0 -> [_ _]
          tunnel: [FALSE w653] -> w650
          event Timeout {
            n297 = event-data() -> ()  [unwired: 1 in, 2 out]
          }
          event "停止": Value Change {
            n298 = event-data() -> ("NewVal"=w654:bool)  [unwired: 1 in, 1 out]
            n299 = case shown="真" w654 {
              selector: w654 -> [_ w656]
              tunnel: [FALSE w656] -> w653
              frame False {
              }
              frame True {
                n300 = local write "开始/暂停"(w656) -> ()
                "停止循环" <- w656
              }
            }
          }
        }
      }
    }
    n301 = local read "Recording"() -> (w643:bool)
    n302 = case shown="真" "热图" {
      tunnel: w641 -> [_ w665]
      tunnel: w635 -> [w657 w663]
      tunnel: [w657 w662] -> w638
      tunnel: w640 -> [_ w660]
      tunnel: w639 -> [_ w659]
      frame False {
      }
      frame True {
        w661 = T4 4 items=["Grayscale (U8)", "Grayscale (I16)", "Grayscale (SGL)", "Complex (CSG)", "RGB (U32)", "HSL (U32)", "RGB (U64)", "Grayscale (U16)"] ("Image Type")
        n303 = call "IMAQ Copy"("Image Dst"=w665, "Image Src"=w663) -> ("Image Dst Out"=w664:T1)  [unwired: 4 in, 1 out]
        n304 = call "IMAQ Divide"("Image Src A"=w664, "Constant"=sgl 256.0, "Image Dst"=w664) -> ("Image Dst Out"=w658:T1)  [unwired: 4 in, 1 out]
        n305 = call "IMAQ Cast Image"("Image Type"=w661, "Lookup Table"=w659, "Image Dst"=w660, "Image Src"=w658) -> ("Image Dst Out"=w662:T1)  [unwired: 6 in, 1 out]
      }
    }
    "Image 2" <- w638
    n306 = Get Queue Status(queue=w630) -> (queue out=w629:refnum<queue>, # elements in queue=→"队列中元素数量":i32)  [unwired: 2 in, 6 out]
    n307 = case shown="真" w643 {
      tunnel: w629 -> [_ w673]
      tunnel: w635 -> [_ w680]
      tunnel: w636 -> [_ w679]
      tunnel: w634 -> [_ w669]
      tunnel: [0 w675] -> w633
      tunnel: w631 -> [_ w670]
      tunnel: [u32[][] [] w672] -> w632
      frame False {
      }
      frame True {
        n308 = call "IMAQ Copy"("Image Dst"=w679, "Image Src"=w680) -> ("Image Dst Out"=w678:T1)  [unwired: 4 in, 1 out]
        n309 = local read "FrameBin"() -> (w674:i32)
        n310 = call "IMAQ ImageToArray"("Image"=w678) -> ("Image Pixels (I16)"=w671:i16[][])  [unwired: 3 in, 4 out]
        n311 = Increment(x=w669) -> (x+1=w676:i32)
        n312 = Greater Or Equal?(x=w674, y=w676) -> (x >= y?=w677:bool)
        n313 = case shown="假" w677 {
          tunnel: w676 -> [_ w691]
          tunnel: [0 w691] -> w675
          tunnel: w673 -> [w685 _]
          tunnel: [u32[][] [] w688] -> w672
          tunnel: w671 -> [w684 w690]
          tunnel: w670 -> [w683 w689]
          tunnel: w669 -> [_ w687]
          frame False {
            n314 = Add(x=w684, y=w683) -> (x+y=w682:u32[][])
            n315 = Enqueue Element(queue=w685, element=w682) -> ()  [unwired: 2 in, 3 out]
          }
          frame True {
            n316 = case shown="0" w687 {
              tunnel: w690 -> [w692 w695]
              tunnel: w689 -> [_ w694]
              tunnel: [w692 w693] -> w688
              frame 0 {
              }
              frame 1, Default {
                n317 = Add(x=w695, y=w694) -> (x+y=w693:u32[][])
              }
            }
          }
        }
      }
    }
    n318 = local read "停止循环"() -> (w642:bool)
    n319 = call <vilib>:"Wait For Frame.vi"("error in (no error)"=w648, "Timeout (mS)"=u32 5000, "RefBrdIn"=w647) -> ("error out"=w649:errorcluster, "RefBrdOut"=w646:u32)  [unwired: 7 in]
    n320 = node-c288() -> ()  [unwired: 1 in, 1 out]
  }
  n321 = local write "Stimuli"(w51) -> ()
  n322 = node-c288(w48) -> ()  [unwired: 1 out]
  n323 = call <vilib>:"Stop.vi"("error in (no error)"=w39, "Image In"=w44, "RefBrdIn"=w26) -> ("error out"=w40:errorcluster, "Image"=w43:T1, "RefBrdOut"=w25:u32)  [unwired: 6 in]
  n324 = call <vilib>:"Cleanup.vi"("error in (no error)"=w40, "Image In"=w43, "RefBrdIn"=w25) -> ("error out"=w41:errorcluster, "Image"=w42:T1, "RefBrdOut"=w24:u32)  [unwired: 6 in]
  n325 = call <vilib>:"Close.vi"("error in (no error)"=w41, "RefBrdIn"=w24) -> ("error out"=w23:errorcluster)  [unwired: 8 in, 1 out]
  n326 = call "Imaq Dispose"("Image"=w42, "error in (no error)"=w23) -> ()  [unwired: 4 in, 1 out]
